vi "NextLine.vi"(1 "Image Settings":T1={"Start Position (µm)"={"x"=0.0, "y"=0.0, "z"=0.0}, "End Position (µm)"={"x"=10.0, "y"=10.0, "z"=0.0}, "Image Resolution (nm/pixel)"={"x"=50.0, "y"=50.0, "z"=100.0}, "Image Size (µm)"={"x"=10.0, "y"=10.0, "z"=0.0}, "Image Size (pixel)"={"x"=50, "y"=50, "z"=0}, "Time Resolution\n(ms/pixel)"=7.0, "1st Axis"=0, "2nd Axis"=1, "Retrace"=FALSE, "Estimated Time"=""} {"2nd Axis" items=["x", "y", "z"]; "1st Axis" items=["x", "y", "z"]; "Time Resolution\n(ms/pixel)" format="%.2f"; "Image Resolution (nm/pixel)"."z" format="%.2f"; "Image Resolution (nm/pixel)"."y" format="%.2f"; "Image Resolution (nm/pixel)"."x" format="%.2f"; "Image Size (µm)"."z" format="%.2f"; "Image Size (µm)"."y" format="%.2f"; "Image Size (µm)"."x" format="%.2f"; "End Position (µm)"."z" format="%.2f"; "End Position (µm)"."y" format="%.2f"; "End Position (µm)"."x" format="%.2f"; "Start Position (µm)"."z" format="%.2f"; "Start Position (µm)"."y" format="%.2f"; "Start Position (µm)"."x" format="%.2f"}) -> (0 "Continue Scan":bool)   [LabVIEW 2009]
uses:
  ImageSettings.ctt
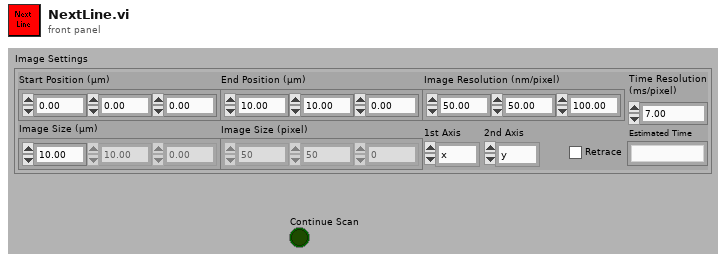
[diagram p1: front panel]
types:
  T1 = typedef "ImageSettings.ctt" = cluster{"Start Position (µm)":cluster{"x":dbl, "y":dbl, "z":dbl}, "End Position (µm)":cluster{"x":dbl, "y":dbl, "z":dbl}, "Image Resolution (nm/pixel)":cluster{"x":dbl, "y":dbl, "z":dbl}, "Image Size (µm)":cluster{"x":dbl, "y":dbl, "z":dbl}, "Image Size (pixel)":cluster{"x":u32, "y":u32, "z":u32}, "Time Resolution\n(ms/pixel)":dbl, "1st Axis":u16, "2nd Axis":u16, "Retrace":bool, "Estimated Time":string}
  T2 = typedef "LineScanStatus.ctt" = cluster{"in line":bool, "line status":cluster{"count":u32, "current":cluster{"x":u32, "y":u32, "z":u32}}, "plane status":cluster{"count":u32, "current":cluster{"x":u32, "y":u32, "z":u32}}, "new line step":cluster{"x":dbl, "y":dbl, "z":dbl}, "new plane step":cluster{"x":dbl, "y":dbl, "z":dbl}}
  T3 = cluster{"current[0]":u32, "current[1]":u32, "current[2]":u32}
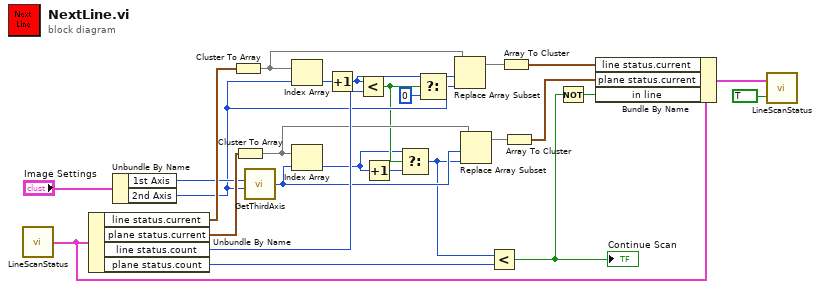
[diagram p0: block diagram]
diagram:
  n1 = call "LineScanStatus.vi"() -> ("Linescan Status (output)"=w22:T2)  [unwired: 2 in]
  n2 = Unbundle By Name(w22) -> ("line status.current"=w26:cluster{"x":u32, "y":u32, "z":u32}, "plane status.current"=w25:cluster{"x":u32, "y":u32, "z":u32}, "line status.count"=w19:u32, "plane status.count"=w7:u32)
  n3 = Unbundle By Name("Image Settings") -> ("1st Axis"=w21:u16, "2nd Axis"=w17:u16)
  n4 = Cluster To Array(cluster=w26) -> (array=w18:u32[])
  n5 = Cluster To Array(cluster=w25) -> (array=w13:u32[])
  n6 = call "GetThirdAxis.vi"("1st Axis"=w17, "2nd Axis"=w21) -> ("3rd Axis"=w12:i32)  [unwired: 2 in]
  n7 = Index Array(array=w18, index=w17) -> (element=w20:u32)
  n8 = Index Array(array=w13, index=w12) -> (element=w10:u32)
  n9 = Increment(x=w20) -> (x+1=w16:u32)
  n10 = Less?(x=w16, y=w19) -> (x < y?=w11:bool)
  n11 = Increment(x=w10) -> (x+1=w9:u32)
  n12 = Select(t=w10, s=w11, f=w9) -> (s? t:f=w8:u32)
  n13 = Select(t=w16, s=w11, f=u32 0) -> (s? t:f=w14:u32)
  n14 = Replace Array Subset(array=w18, new element=w14, index=w17) -> (w6:u32[])
  n15 = Replace Array Subset(array=w13, new element=w8, index=w12) -> (w5:u32[])
  n16 = Less?(x=w8, y=w7) -> (x < y?=w2:bool)
  "Continue Scan" <- w2
  n17 = Array To Cluster(array=w6) -> (cluster=w3:T3)
  n18 = Array To Cluster(array=w5) -> (cluster=w4:T3)
  n19 = Not(x=w2) -> (.not. x?=w1:bool)
  n20 = Bundle By Name(cluster=w22, "line status.current"=w3, "plane status.current"=w4, "in line"=w1) -> (w23:T2)
  n21 = call "LineScanStatus.vi"("Get/Set"=TRUE, "Linescan Status (input)"=w23) -> ()  [unwired: 1 out]
